vi "LevMar.vi"(6 "max iteration":i32=200 caption="nombre max d'itérations", 7 "Target function in":refnum<vi>, 8 "error in (no error)":errorcluster, 9 "Standard Deviation":dbl[](array[numeric]) caption="Écart-type" format="%0.2f", 10 "Y":dbl[](array[numeric]) format="%0.2f", 11 "Initial Guess Coefficients":dbl[](array[numeric]) caption="Coefficients estimés initiaux" format="%0.2f") -> (0 "error out":errorcluster, 1 "Covariance":dbl[][](array[numeric]) format="%0.2f", 2 "Best Fit":dbl[](array[numeric]) caption="Meilleur ajustement" format="%0.2f", 3 "Best Fit Coefficients":dbl[](array[numeric]) caption="Coefficients d'ajustement optimaux" format="%0.2f", 4 "mse":dbl caption="erreur quadratique moyenne" format="%0.4e", 5 "Target function out":refnum<vi>)   [LabVIEW 2009]
doc: "Utilise l'algorithme de Levenberg-Marquardt pour déterminer le jeu de coefficients des moindres carrés qui s'ajuste le mieux à l'ensemble de points de données d'entrée (X,Y), exprimé par une fonction non linéaire y=f(x,a) où a est le jeu de coefficients."
uses:
  <vilib>/Analysis/baseanly.llb/Real Inverse Matrix.vi
  <vilib>/Analysis/NI_AALPro.lvlib
  <vilib>/Analysis/NI_AALBase.lvlib
panel:
  # "Ajustement non-linéaire de Levenberg-Marquardt"
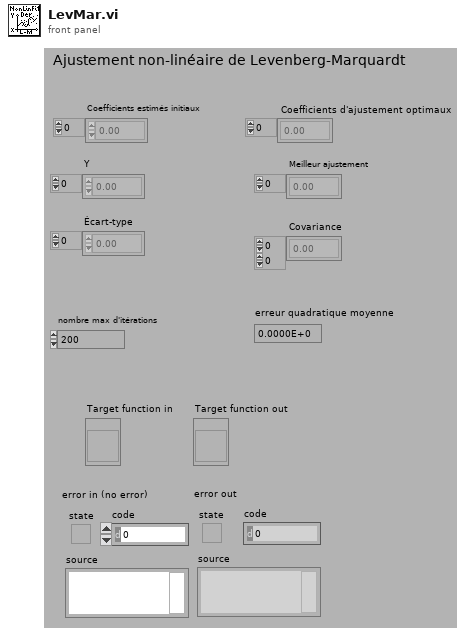
[diagram p1: front panel]
types:
  T1 = typedef "NI_Matrix.lvlib/RealMatrix.ctl" = dbl[][]
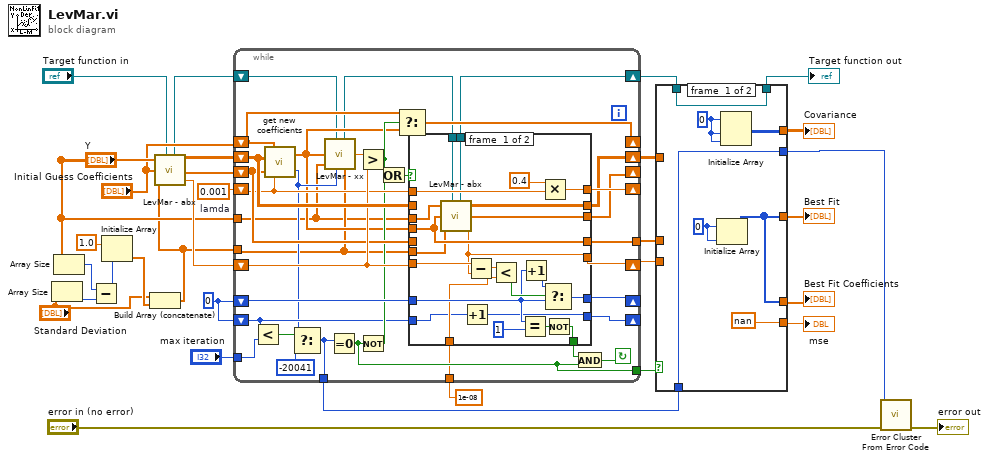
[diagram p0: block diagram]
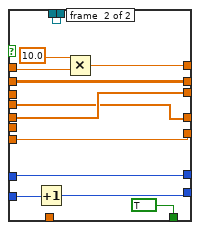
[diagram p2: hidden frame]
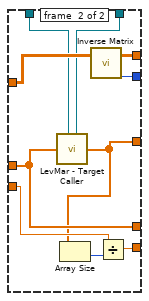
[diagram p3: hidden frame]
diagram:
  w22 = 0
  w31 = 0.001  # lamda
  n1 = Array Size(array="Standard Deviation") -> (size(s)=w14:i32)
  n2 = Array Size(array="Y") -> (size(s)=w15:i32)
  n3 = Subtract(x=w15, y=w14) -> (x-y=w13:i32)
  n4 = Initialize Array(1.0, w13) -> (w12:dbl[])
  n5 = Build Array (concatenate)("Standard Deviation", w12) -> (w8:dbl[])
  n6 = call "LevMar - abx.vi"("Y"="Y", "Target function in"="Target function in", "Coefficients"="Initial Guess Coefficients", "Standard Deviation"=w8) -> ("Target function out"=w6:refnum<vi>, "Alpha"=w32:dbl[][], "Beta"=w30:dbl[], "chiSqr"=w29:dbl)  [unwired: 2 in]
  n7 = while {
    tunnel: "Y" -> [w35]
    tunnel: [w41] -> w17
    tunnel: "max iteration" -> [w42]
    tunnel: w8 -> [w36]
    shift-left: w22 -> [w46]
    shift-right: [w47] -> _
    tunnel: 1e-08 -> [w51]
    tunnel: [w52] -> w24
    tunnel: [w55] -> w27
    shift-left: w22 -> [w59]
    shift-right: [w58] -> _
    shift-left: w29 -> [w60]
    shift-right: [w61] -> w28
    shift-left: w30 -> [w57]
    shift-right: [w39] -> _
    shift-left: w32 -> [w62]
    shift-right: [w63] -> w16
    shift-left: "Initial Guess Coefficients" -> [w40]
    shift-right: [w64] -> _
    shift-left: w31 -> [w56]
    shift-right: [w65] -> _
    shift-right: [w38] -> w5
    shift-left: w6 -> [w34]
    stop <- w54 continue-if-true
    n8 = Less?(x=w46, y=w42) -> (x < y?=w45:bool)
    n9 = call <vilib>:"get new coefficients.vi"("lamda"=w56, "Beta"=w57, "Alpha"=w62, "Coefficients"=w40) -> ("error"=w43:i32, "New Coefficients"=w37:dbl[])
    n10 = Select(t=w43, s=w45, f=-20041) -> (s? t:f=w41:i32)
    n11 = call "LevMar - xx.vi"("Target function in"=w34, "Coefficients"=w37, "Y"=w35, "error"=w43, "Standard Deviation"=w36) -> ("Target function out"=w33:refnum<vi>, "chiSqr"=w66:dbl)  [unwired: 3 in]
    n12 = Equal To 0?(x=w41) -> (x = 0?=w52:bool)
    n13 = Greater?(x=w66, y=w60) -> (0:w49:bool)
    n14 = Not(x=w52) -> (.not. x?=w48:bool)
    n15 = Or(x=w49, y=w48) -> (x .or. y?=w50:bool)
    n16 = Select(t=w40, s=w49, f=w37) -> (s? t:f=w64:dbl[])
    n17 = case shown="False" w50 {
      tunnel: w56 -> [w88 w100]
      tunnel: [w87 w99] -> w65
      tunnel: [w86 w98] -> w63
      tunnel: w62 -> [_ w98]
      tunnel: [w85 w94] -> w39
      tunnel: [w69 w97] -> w61
      tunnel: w60 -> [w84 w97]
      tunnel: w59 -> [w79 w96]
      tunnel: [w80 w96] -> w58
      tunnel: [w76 TRUE] -> w53
      tunnel: w37 -> [w71 w93]
      tunnel: w57 -> [_ w94]
      tunnel: [w71 w93] -> w55
      tunnel: w51 -> [w75 _]
      tunnel: [w73 w92] -> w47
      tunnel: w46 -> [w74 w91]
      tunnel: w36 -> [w70 _]
      tunnel: w35 -> [w72 _]
      tunnel: w33 -> [w68 w90]
      tunnel: [w67 w90] -> w38
      frame #0 {
        n18 = call "LevMar - abx.vi"("Y"=w72, "Target function in"=w68, "Coefficients"=w71, "Standard Deviation"=w70) -> ("Target function out"=w67:refnum<vi>, "Alpha"=w86:dbl[][], "Beta"=w85:dbl[], "chiSqr"=w69:dbl)  [unwired: 2 in]
        n19 = Increment(x=w74) -> (x+1=w73:i32)
        n20 = Subtract(x=w84, y=w69) -> (x-y=w83:dbl)
        n21 = Less?(x=w83, y=w75) -> (x < y?=w82:bool)
        n22 = Equal?(x=w79, y=1) -> (x = y?=w77:bool)
        n23 = Increment(x=w79) -> (x+1=w81:i32)
        n24 = Multiply(x=0.4, y=w88) -> (x*y=w87:dbl)
        n25 = Select(t=w81, s=w82, f=w79) -> (s? t:f=w80:i32)
        n26 = Not(x=w77) -> (.not. x?=w76:bool)
      }
      frame #1 {
        n27 = Increment(x=w91) -> (x+1=w92:i32)
        n28 = Multiply(x=10.0, y=w100) -> (x*y=w99:dbl)
      }
    }
    n29 = And(x=w53, y=w52) -> (x .and. y?=w54:bool)
  }
  n30 = case shown="True" w24 {
    tunnel: w27 -> [_ w116]
    tunnel: [w106 w116] -> w26
    tunnel: [nan w118] -> w25
    tunnel: [w106 w111] -> w19
    tunnel: w28 -> [_ w112]
    tunnel: [w104 w115] -> w18
    tunnel: [w103 w114] -> w1
    tunnel: w17 -> [w103 _]
    tunnel: w16 -> [_ w113]
    tunnel: w5 -> [w102 w110]
    tunnel: [w102 w109] -> w4
    frame #0 {
      w105 = 0
      w108 = 0
      n31 = Initialize Array(w108, w108) -> (w106:i32[])
      n32 = Initialize Array(w105, w105, w105) -> (w104:i32[][])
    }
    frame #1 {
      n33 = call "LevMar - Target Caller.vi"("A"=w116, "Target Function in"=w110) -> ("Target Function out"=w109:refnum<vi>, "F"=w111:dbl[])
      n34 = Array Size(array=w111) -> (size(s)=w117:i32)
      n35 = call-poly <vilib>:"Inverse Matrix.vi"("Input Matrix"=w113) -> ("error"=w114:i32, "Inverse Matrix"=w115:T1)  [unwired: 1 in]
      n36 = Divide(x=w112, y=w117) -> (x/y=w118:dbl)
    }
  }
  "mse" <- w25
  "Best Fit Coefficients" <- w26
  "Best Fit" <- w19
  "Covariance" <- w18
  "Target function out" <- w4
  n37 = call <vilib>:"Error Cluster From Error Code.vi"("error in (no error)"="error in (no error)", "error code (0)"=w1) -> ("error out"=→"error out":errorcluster)  [unwired: 7 in]
